vi "Fill VCluster.vi"(8 "error in (no error)":errorcluster, 10 "Cluster In":variant, 11 "LV Argument Parser in":refnum<class "LV Argument Parser.lvclass">) -> (0 "error out":errorcluster, 2 "Filled Cluster Out":variant, 3 "LV Argument Parser out":refnum<class "LV Argument Parser.lvclass">)   [LabVIEW 2023, in "LV ArgParse.lvlib" / "LV Argument Parser.lvclass"]
uses:
  LV Argument Parser.lvclass
  LV Argument Parser.lvclass/LV Argument Parser.ctl
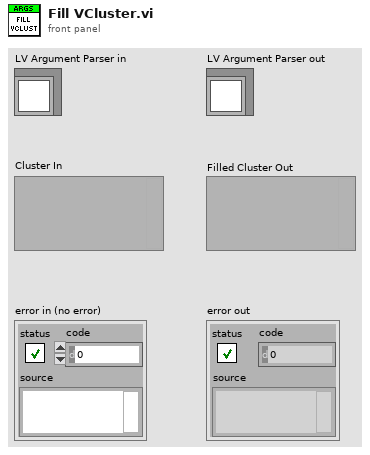
[diagram p1: front panel]
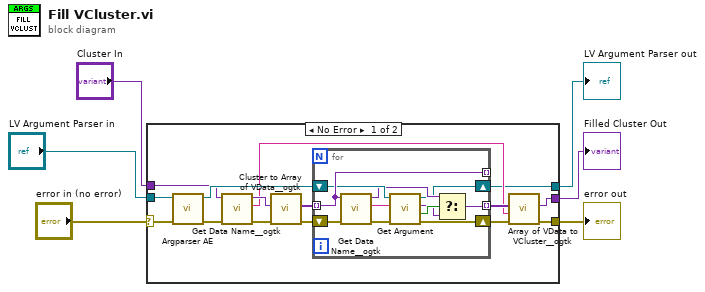
[diagram p0: block diagram]
diagram:
  n1 = case shown="No Error" "error in (no error)" {
    selector: "error in (no error)" -> [w21 w35]
    tunnel: [w8 w35] -> w5
    tunnel: [w7 w34] -> w3
    tunnel: "LV Argument Parser in" -> [w20 w34]
    tunnel: "Cluster In" -> [w13 w33]
    tunnel: [w9 w33] -> w1
    frame No Error {
      n2 = call "Argparser AE.vi"("error in (no error)"=w21, "LV Argument Parser in"=w20) -> ("error out"=w19:errorcluster, "LV Argument Parser out"=w16:refnum<class "LV Argument Parser.lvclass">)  [unwired: 8 in]
      n3 = call <userlib>:"Get Data Name__ogtk.vi"("error in (no error)"=w19, "Data"=w13) -> ("error out"=w14:errorcluster, "Data Name"=w11:string, "Data dup"=w12:variant)  [unwired: 7 in]
      n4 = call <userlib>:"Cluster to Array of VData__ogtk.vi"("error in (no error)"=w14, "Cluster"=w12) -> ("error out"=w17:errorcluster, "Array of VData"=w18:variant[])  [unwired: 8 in]
      n5 = for {
        tunnel: [w32] -> _ mode=indexing
        tunnel: w18 -> [w32] mode=indexing
        tunnel: [w24] -> w15 mode=indexing
        shift-right: [w23] -> w10
        shift-left: w17 -> [w31]
        shift-right: [w22] -> w7
        shift-left: w16 -> [w28]
        n6 = call <userlib>:"Get Data Name__ogtk.vi"("error in (no error)"=w31, "Data"=w32) -> ("error out"=w30:errorcluster, "Data Name"=w29:string, "Data dup"=w25:variant)  [unwired: 7 in]
        n7 = call "Get Argument.vi"("error in (no error)"=w30, "Name"=w29, "LV Argument Parser in"=w28) -> ("error out"=w23:errorcluster, "key not found?"=w27:bool, "element"=w26:variant, "LV Argument Parser out"=w22:refnum<class "LV Argument Parser.lvclass">)  [unwired: 5 in]
        n8 = Select(t=w25, s=w27, f=w26) -> (s? t:f=w24:variant)
      }
      n9 = call <userlib>:"Array of VData to VCluster__ogtk.vi"("error in (no error)"=w10, "Cluster Name"=w11, "Array"=w15) -> ("error out"=w8:errorcluster, "VCluster"=w9:variant)  [unwired: 7 in]
    }
    frame Error {
    }
  }
  "error out" <- w5
  "LV Argument Parser out" <- w3
  "Filled Cluster Out" <- w1
